vi "Set InitializationVI Path.vi"(8 "error in (no error)":errorcluster, 10 "Path in":string, 11 "Project XML Editor in":refnum<class "Project XML Editor.lvclass">) -> (0 "error out":errorcluster, 3 "Project XML Editor out":refnum<class "Project XML Editor.lvclass">)   [LabVIEW 2019, in "LVLIBP CD XML Updater.lvlib" / "Project XML Editor.lvclass"]
uses:
  Project XML Editor.lvclass
  <vilib>/xml/Close Reference(Node).vi
  <vilib>/xml/NI_XML.lvlib
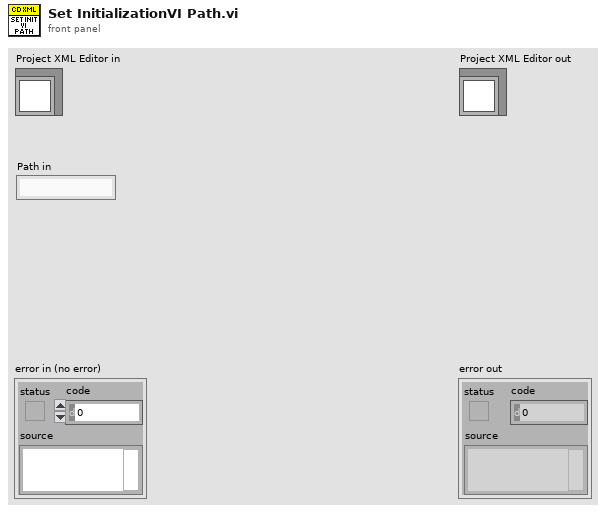
[diagram p1: front panel]
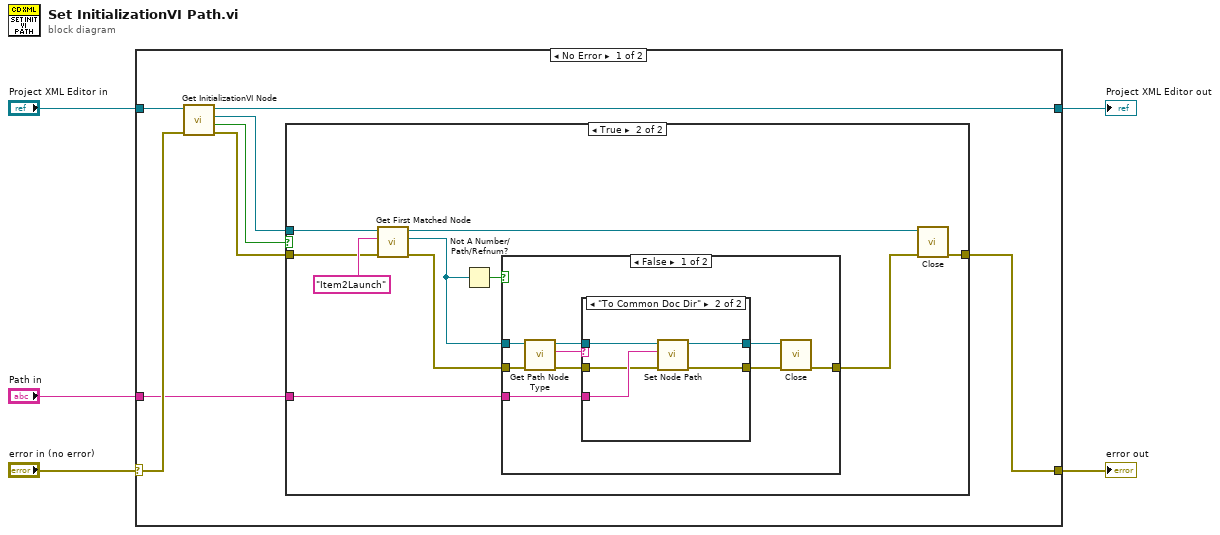
[diagram p0: block diagram]
diagram:
  n1 = case shown="No Error" "error in (no error)" {
    selector: "error in (no error)" -> [w7 w43]
    tunnel: [w13 w43] -> w4
    tunnel: [w11 w42] -> w2
    tunnel: "Project XML Editor in" -> [w12 w42]
    tunnel: "Path in" -> [w6 _]
    frame No Error {
      n2 = call "Get InitializationVI Node.vi"("error in (no error)"=w7, "Project XML Editor in"=w12) -> ("error out"=w8:errorcluster, "Found?"=w9:bool, "Node ref out"=w10:refnum<k20>, "Project XML Editor out"=w11:refnum<class "Project XML Editor.lvclass">)  [unwired: 6 in]
      n3 = case shown="True" w9 {
        tunnel: w10 -> [_ w24]
        tunnel: w8 -> [w14 w21]
        tunnel: [w14 w19] -> w13
        tunnel: w6 -> [_ w16]
        frame False {
        }
        frame True {
          n4 = call <vilib>:"Get First Matched Node.vi"("error in (no error)"=w21, "XPath expression"="Item2Launch", "node in"=w24) -> ("error out"=w20:errorcluster, "node result"=w18:refnum<k20>, "node out"=w22:refnum<k20>)  [unwired: 6 in]
          n5 = Not A Number/Path/Refnum?(number/path/refnum=w18) -> (NaN/Path/Refnum?=w17:bool)
          n6 = case shown="False" w17 {
            tunnel: w20 -> [w32 w41]
            tunnel: [w26 w41] -> w15
            tunnel: w18 -> [w33 _]
            tunnel: w16 -> [w29 _]
            frame False {
              n7 = call "Get Path Node Type.vi"("error in (no error)"=w32, "Node ref in"=w33) -> ("error out"=w31:errorcluster, "Path Type out"=w25:string, "Node ref out"=w30:refnum<k20>)  [unwired: 6 in, 1 out]
              n8 = case shown="\"To Common Doc Dir\"" w25 {
                tunnel: w31 -> [w35 w38]
                tunnel: w30 -> [w34 w40]
                tunnel: w29 -> [_ w39]
                tunnel: [w35 w37] -> w27
                tunnel: [w34 w36] -> w28
                frame "Other", Default {
                }
                frame "To Common Doc Dir" {
                  n9 = call "Set Node Path.vi"("error in (no error)"=w38, "Path in"=w39, "Node ref in"=w40) -> ("error out"=w37:errorcluster, "Node ref out"=w36:refnum<k20>)  [unwired: 6 in, 1 out]
                }
              }
              n10 = call-poly <vilib>:"Close.vi"("error in (no error)"=w27, "node"=w28) -> ("error out"=w26:errorcluster)  [unwired: 7 in]
            }
            frame True {
            }
          }
          n11 = call-poly <vilib>:"Close.vi"("error in (no error)"=w15, "node"=w22) -> ("error out"=w19:errorcluster)  [unwired: 7 in]
        }
      }
    }
    frame Error {
    }
  }
  "error out" <- w4
  "Project XML Editor out" <- w2
